vi "JTAG Config.vi"(8 "error in (no error)":errorcluster, 11 "Function":u16(ring)=5 items=["Initialize COMMs", "Release COMMs", "Initialize Variables", "Select 1MHz DCO", "Select 8MHz DCO", "Standard Startup"]) -> (0 "error out":errorcluster)   [LabVIEW 2010]
panel:
  out "PC start address":u16=14304 format="%04x"
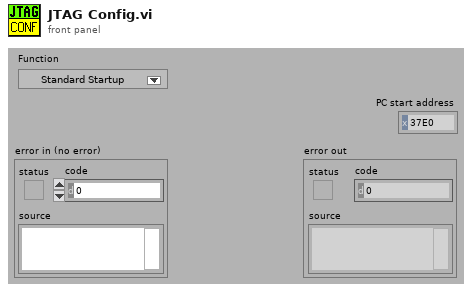
[diagram p1: front panel]
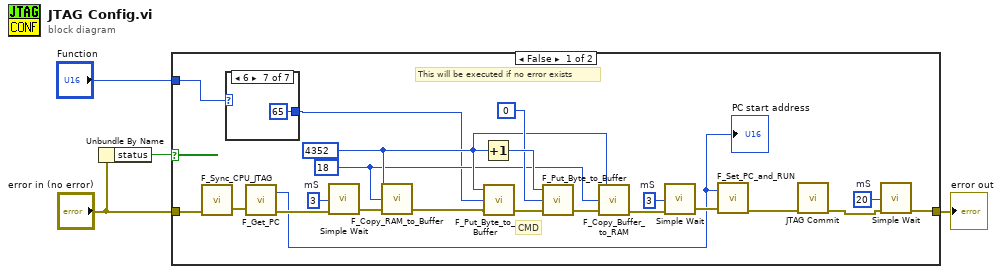
[diagram p0: block diagram]
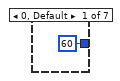
[diagram p2: hidden frame]
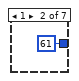
[diagram p3: hidden frame]
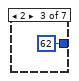
[diagram p4: hidden frame]
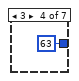
[diagram p5: hidden frame]
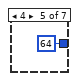
[diagram p6: hidden frame]
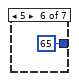
[diagram p7: hidden frame]
diagram:
  n1 = Unbundle By Name("error in (no error)") -> ("status"=w3:bool)
  n2 = case shown="False" w3 {
    tunnel: [w5 w34] -> w4
    tunnel: "error in (no error)" -> [w11 w34]
    tunnel: "Function" -> [w14 _]
    frame False {
      w7 = u32 20  # mS
      w21 = u32 3  # mS
      w22 = u32 3  # mS
      w17 = u16 18
      w18 = u16 4352
      # "CMD"
      # "This will be executed if no error exists"
      n3 = call "F_Sync_CPU_JTAG.vi"("error in (no error)"=w11) -> ("error out"=w10:errorcluster)  [unwired: 1 in, 1 out]
      n4 = case shown="6" w14 {
        tunnel: [60 61 62 63 64 65 65] -> w12
        frame 0, Default {
        }
        frame 1 {
        }
        frame 2 {
        }
        frame 3 {
        }
        frame 4 {
        }
        frame 5 {
        }
        frame 6 {
        }
      }
      n5 = call "F_Get_PC.vi"("error in (no error)"=w10) -> ("error out"=w9:errorcluster, "Program Counter"=w8:u16)  [unwired: 1 in]
      "PC start address" <- w8
      n6 = call "Simple Wait.vi"("mS"=w22, "error in"=w9) -> ("error out"=w19:errorcluster)  [unwired: 12 in, 1 out]
      n7 = call "F_Copy_RAM_to_Buffer.vi"("error in (no error)"=w19, "Block size to be copied"=w17, "RAM start address"=w18) -> ("error out"=w16:errorcluster)  [unwired: 2 in]
      n8 = Increment(x=w18) -> (x+1=w25:u16)
      n9 = call "F_Put_Byte_to_Buffer.vi"("error in (no error)"=w16, "New value"=w12, "Address of byte to be updated"=w18) -> ("error out"=w26:errorcluster)  [unwired: 2 in]
      n10 = call "F_Put_Byte_to_Buffer.vi"("error in (no error)"=w26, "New value"=u16 0, "Address of byte to be updated"=w25) -> ("error out"=w23:errorcluster)  [unwired: 2 in]
      n11 = call "F_Copy_Buffer_to_RAM.vi"("error in (no error)"=w23, "Block size to be copied"=w17, "Buffer start address"=w18) -> ("error out"=w20:errorcluster)  [unwired: 2 in]
      n12 = call "Simple Wait.vi"("mS"=w21, "error in"=w20) -> ("error out"=w15:errorcluster)  [unwired: 12 in, 1 out]
      n13 = call "F_Set_PC_and_RUN.vi"("error in (no error)"=w15, "PC start address"=w8) -> ("error out"=w13:errorcluster)  [unwired: 1 in]
      n14 = call "JTAG Commit.vi"("error in (no error)"=w13) -> ("error out"=w6:errorcluster)  [unwired: 10 in]
      n15 = call "Simple Wait.vi"("mS"=w7, "error in"=w6) -> ("error out"=w5:errorcluster)  [unwired: 12 in, 1 out]
    }
    frame True {
      # "Error exists, skip all functions"
    }
  }
  "error out" <- w4
